vi "CreateNewSystemDefinition.vi"(8 "error in (no error)":errorcluster, 10 "System Definition Name":string, 11 "VeriStandScriptingTestCase in":refnum<class "VeriStandScriptingTestCase.lvclass">) -> (0 "error out":errorcluster, 3 "VeriStandScriptingTestCase out":refnum<class "VeriStandScriptingTestCase.lvclass">)   [LabVIEW 2027, in "VeriStandScriptingTestCase.lvclass"]
uses:
  VeriStandScriptingTestCase.lvclass
  VeriStandTestUtilities/VeriStandTestUtilities.lvlib
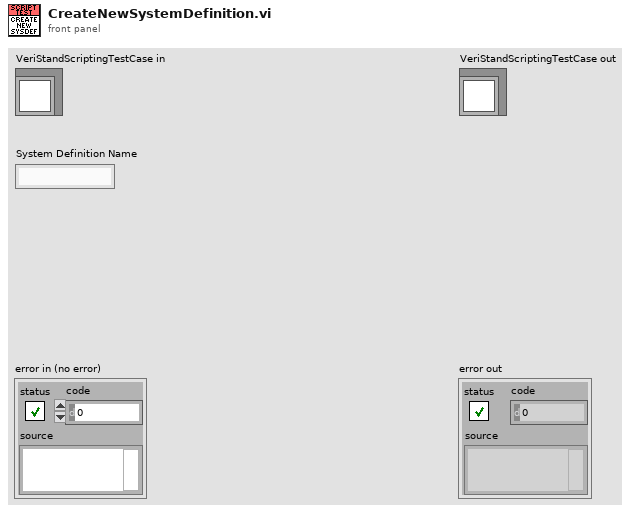
[diagram p1: front panel]
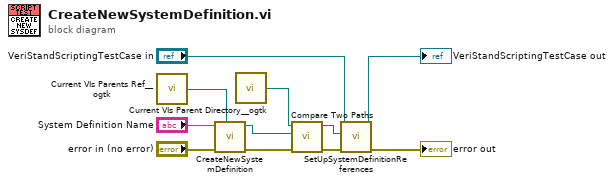
[diagram p0: block diagram]
diagram:
  n1 = call <userlib>:"Current VIs Parents Ref__ogtk.vi"() -> ("Calling VI's Reference"=w1:refnum<vi>)  [unwired: 2 in]
  n2 = call "CreateNewSystemDefinition.vi"("test VI ref"=w1, "error in"="error in (no error)", "System Definition Name"="System Definition Name") -> ("error out"=w9:errorcluster, "System Definition Path"=w8:path)  [unwired: 7 in]
  n3 = call <userlib>:"Current VIs Parent Directory__ogtk.vi"() -> ("Parent Directory (+ Relative)"=w7:path)  [unwired: 5 in]
  n4 = call <vilib>:"Compare Two Paths.vi"("error in (no error)"=w9, "Path 2"=w8, "Path 1"=w7) -> ("error out"=w6:errorcluster, "Relative Path from 1 to 2"=w4:path)  [unwired: 5 in, 2 out]
  n5 = call "SetUpSystemDefinitionReferences.vi"("error in"=w6, "Relative Path to SysDef"=w4, "VeriStandScriptingTestCase in"="VeriStandScriptingTestCase in") -> ("error out"=→"error out":errorcluster, "VeriStandScriptingTestCase out"=→"VeriStandScriptingTestCase out":refnum<class "VeriStandScriptingTestCase.lvclass">)  [unwired: 7 in]
